vi "ResponseStringToSignalCluster(obj).vi"(8 "error in (no error)":errorcluster, 11 "T560Output in":refnum<class "T560Output.lvclass">) -> (0 "error out":errorcluster, 3 "T560Output out":refnum<class "T560Output.lvclass">)   [LabVIEW 2020, in "T560Output.lvclass"]
doc: "Update the value of 'T560Output.Signal' cluster by converting the 'T560Output.Response' string"
uses:
  T560Output.lvclass
  C:/GEECS/Developers Version/source/Device Drivers/Highland T564 DDG/SupportLibraries/DeviceSpecific/HighlandT560Lib/T560ChannelClass/T560Channel.lvclass
  T560Output.lvclass/T560Output.ctl
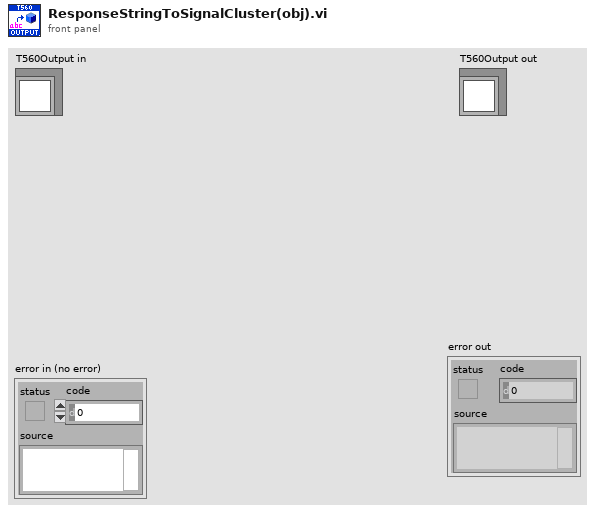
[diagram p1: front panel]
types:
  T1 = typedef "ChannelPolarity.ctl" = enum16{"Direct", "Inverted"}
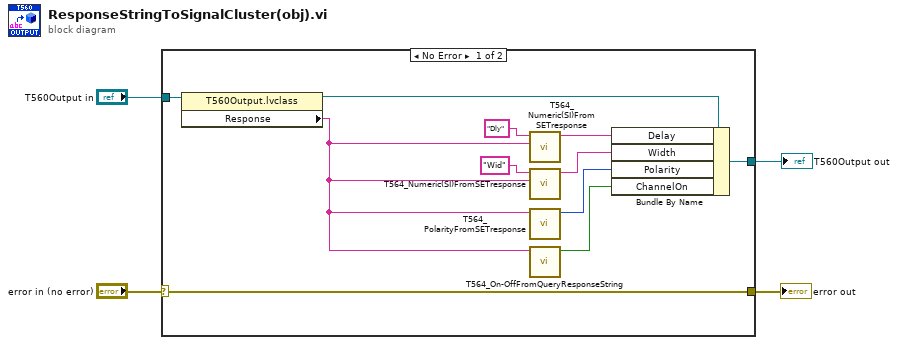
[diagram p0: block diagram]
diagram:
  n1 = case shown="No Error" "error in (no error)" {
    selector: "error in (no error)" -> [w5 w16]
    tunnel: "T560Output in" -> [w13 w17]
    tunnel: [w7 w17] -> w3
    tunnel: [w5 w16] -> w1
    frame No Error {
      n2 = property class="T560Output.lvclass"(reference=w13) -> (reference out=w6:refnum<class "T560Output.lvclass">, "Response"=w8:string)  [unwired: 1 in, 1 out]
      n3 = call "T564_Numeric(SI)FromSETresponse.vi"("StringIn"=w8, "Prefix"="Dly" ("regular expression")) -> ("SI_String"=w12:string)  [unwired: 9 in]
      n4 = call "T564_Numeric(SI)FromSETresponse.vi"("StringIn"=w8, "Prefix"="Wid" ("regular expression")) -> ("SI_String"=w11:string)  [unwired: 9 in]
      n5 = call "T564_PolarityFromSETresponse.vi"("String"=w8) -> ("Polarity"=w10:T1)  [unwired: 10 in]
      n6 = call "T564_On-OffFromQueryResponseString.vi"("String"=w8) -> ("ChannelON?"=w9:bool)  [unwired: 10 in]
      n7 = Bundle By Name(cluster=w6, "Delay"=w12, "Width"=w11, "Polarity"=w10, "ChannelOn"=w9) -> (w7:refnum<class "T560Output.lvclass">)
    }
    frame Error {
    }
  }
  "error out" <- w1
  "T560Output out" <- w3
